vi "LedRingSubVI.vi"(8 "error in (no error)":errorcluster, 9 "Enum":enum16{"Idle", "Off", "Block", "Access"}(ring), 10 "VISA resource name in":refnum<visa-resource-name>, 11 "Boolean in":refnum<vi>) -> (0 "error out":errorcluster, 3 "VISA Refnum out":refnum<visa-resource-name>)   [LabVIEW 2024]
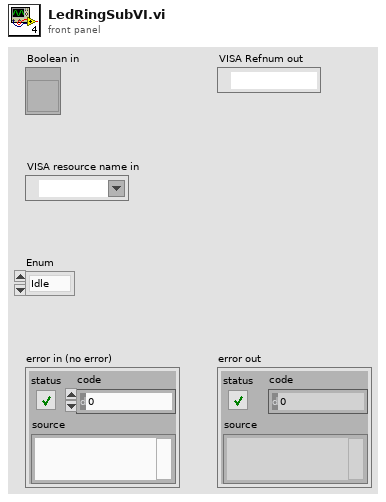
[diagram p1: front panel]
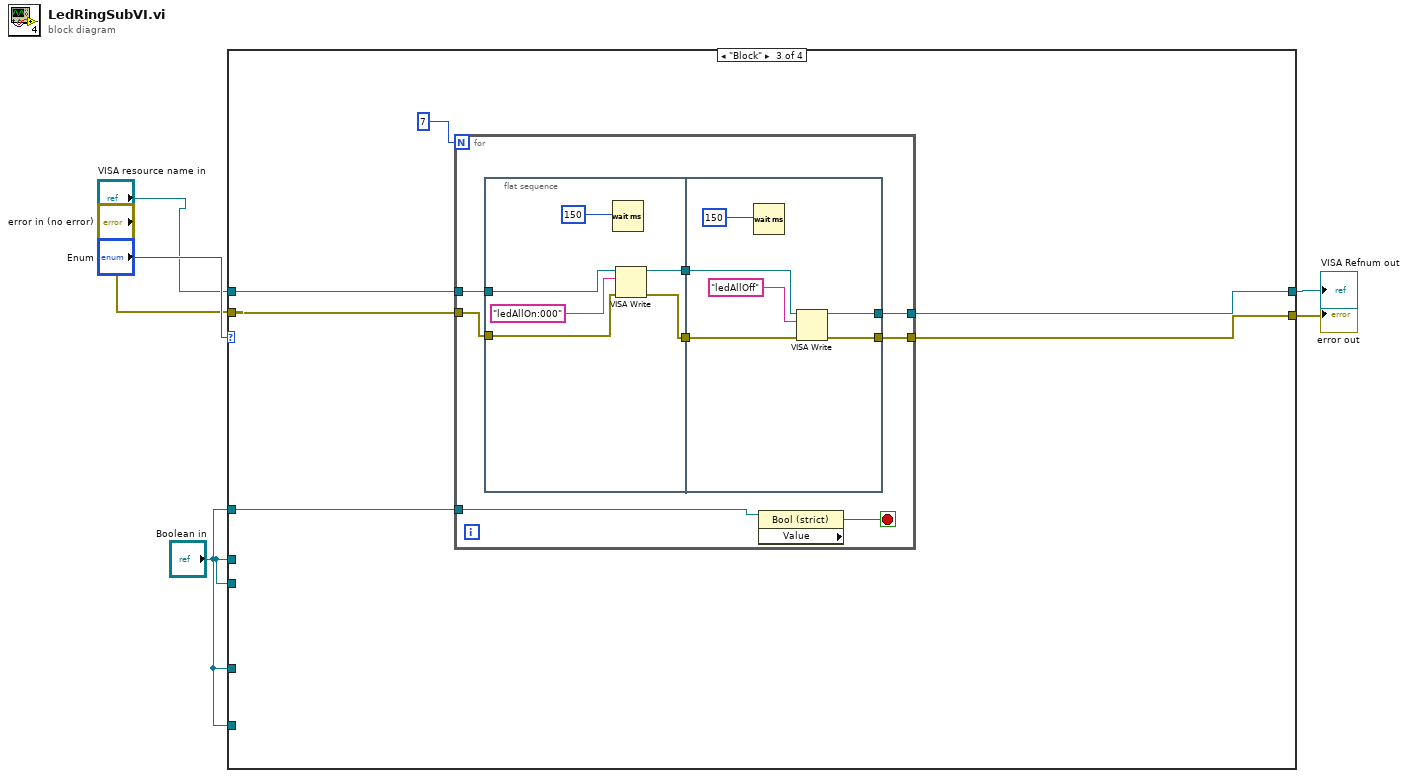
[diagram p0: block diagram]
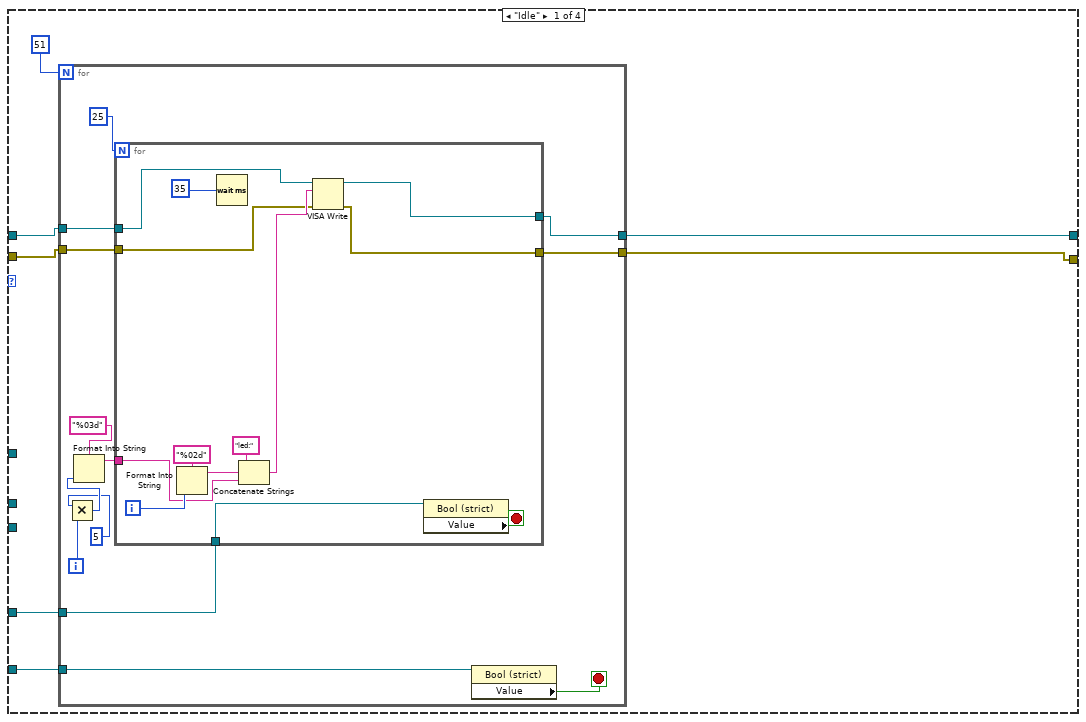
[diagram p2: hidden frame]
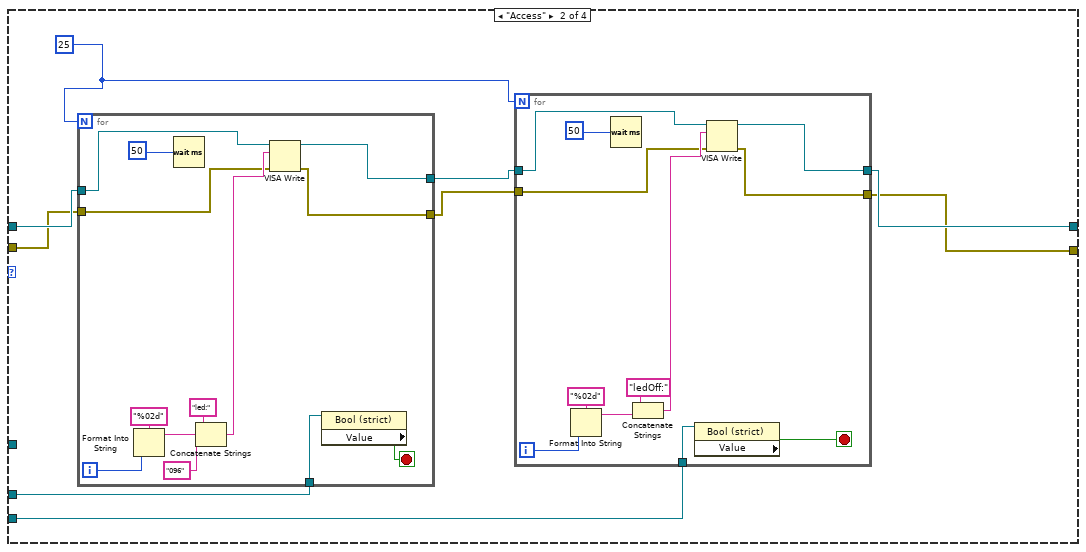
[diagram p3: hidden frame]
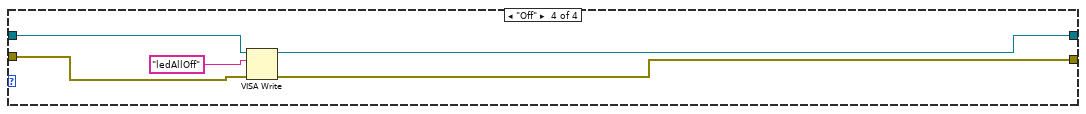
[diagram p4: hidden frame]
diagram:
  n1 = case shown="\"Access\"" "Enum" {
    tunnel: "VISA resource name in" -> [w12 w45 w78 w103]
    tunnel: "error in (no error)" -> [w13 w44 w77 w102]
    tunnel: [w10 w43 w76 w101] -> w5
    tunnel: [w9 w42 w75 w100] -> w4
    tunnel: "Boolean in" -> [w8 _ _ _]
    tunnel: "Boolean in" -> [w7 _ _ _]
    tunnel: "Boolean in" -> [_ w41 _ _]
    tunnel: "Boolean in" -> [_ w40 _ _]
    tunnel: "Boolean in" -> [_ _ w74 _]
    frame "Idle" {
      n2 = for {
        N: 51 -> [_]
        tunnel: w13 -> [w26]
        tunnel: w12 -> [w25]
        tunnel: [w21] -> w10
        tunnel: [w20] -> w9
        tunnel: w8 -> [w15]
        tunnel: w7 -> [w14]
        i -> [w19]
        stop <- w16 stop-if-true
        n3 = Multiply(x=5, y=w19) -> (x*y=w18:i32)
        n4 = Format Into String(format string="%03d", w18) -> (resulting string=w22:string)  [unwired: 2 in, 1 out]
        n5 = for {
          N: 25 -> [_]
          tunnel: w26 -> [w32]
          tunnel: w25 -> [w33]
          tunnel: [w34] -> w20
          tunnel: [w35] -> w21
          tunnel: w22 -> [w29]
          tunnel: w15 -> [w27]
          i -> [w38]
          stop <- w28 stop-if-true
          n6 = Format Into String(format string="%02d", w38) -> (resulting string=w30:string)  [unwired: 2 in, 1 out]
          n7 = Wait (ms)(milliseconds to wait=u32 35 ("millisecond multiple")) -> ()  [unwired: 1 out]
          n8 = Concatenate Strings("led:", w30, w29) -> (w36:string)
          n9 = VISA Write(VISA resource name=w33, write buffer=w36, error in (no error)=w32) -> (VISA resource name out=w35:refnum<visa-resource-name>, error out=w34:errorcluster)  [unwired: 1 out]
          n10 = property class="Bool (strict)"(reference=w27) -> ("Value"=w28:bool)  [unwired: 1 in, 2 out]
        }
        n11 = property class="Bool (strict)"(reference=w14) -> ("Value"=w16:bool)  [unwired: 1 in, 2 out]
      }
    }
    frame "Access" {
      w46 = 25
      n12 = for {
        N: w46 -> [_]
        tunnel: w44 -> [w65]
        tunnel: w45 -> [w66]
        tunnel: [w67] -> w47
        tunnel: [w68] -> w48
        tunnel: w41 -> [w61]
        i -> [w72]
        stop <- w62 stop-if-true
        n13 = Format Into String(format string="%02d", w72) -> (resulting string=w63:string)  [unwired: 2 in, 1 out]
        n14 = Wait (ms)(milliseconds to wait=u32 50 ("millisecond multiple")) -> ()  [unwired: 1 out]
        n15 = Concatenate Strings("led:", w63, "096") -> (w69:string)
        n16 = VISA Write(VISA resource name=w66, write buffer=w69, error in (no error)=w65) -> (VISA resource name out=w68:refnum<visa-resource-name>, error out=w67:errorcluster)  [unwired: 1 out]
        n17 = property class="Bool (strict)"(reference=w61) -> ("Value"=w62:bool)  [unwired: 1 in, 2 out]
      }
      n18 = for {
        N: w46 -> [_]
        tunnel: w47 -> [w53]
        tunnel: w48 -> [w54]
        tunnel: [w55] -> w42
        tunnel: [w56] -> w43
        tunnel: w40 -> [w49]
        i -> [w59]
        stop <- w50 stop-if-true
        n19 = Format Into String(format string="%02d", w59) -> (resulting string=w51:string)  [unwired: 2 in, 1 out]
        n20 = Wait (ms)(milliseconds to wait=u32 50 ("millisecond multiple")) -> ()  [unwired: 1 out]
        n21 = Concatenate Strings("ledOff:", w51) -> (w57:string)
        n22 = property class="Bool (strict)"(reference=w49) -> ("Value"=w50:bool)  [unwired: 1 in, 2 out]
        n23 = VISA Write(VISA resource name=w54, write buffer=w57, error in (no error)=w53) -> (VISA resource name out=w56:refnum<visa-resource-name>, error out=w55:errorcluster)  [unwired: 1 out]
      }
    }
    frame "Block" {
      n24 = for {
        N: 7 -> [_]
        tunnel: w78 -> [w85]
        tunnel: w77 -> [w84]
        tunnel: [w83] -> w76
        tunnel: [w82] -> w75
        tunnel: w74 -> [w80]
        stop <- w81 stop-if-true
        n25 = flat-sequence {
          tunnel: [w91] -> w87
          tunnel: [w90] -> w86
          tunnel: w85 -> [w89]
          tunnel: w84 -> [w88]
          tunnel: w87 -> [w98]
          tunnel: w86 -> [w97]
          tunnel: [w96] -> w83
          tunnel: [w95] -> w82
          frame #0 {
            n26 = Wait (ms)(milliseconds to wait=u32 150 ("millisecond multiple")) -> ()  [unwired: 1 out]
            n27 = VISA Write(VISA resource name=w89, write buffer="ledAllOn:000", error in (no error)=w88) -> (VISA resource name out=w91:refnum<visa-resource-name>, error out=w90:errorcluster)  [unwired: 1 out]
          }
          frame #1 {
            n28 = Wait (ms)(milliseconds to wait=u32 150 ("millisecond multiple")) -> ()  [unwired: 1 out]
            n29 = VISA Write(VISA resource name=w98, write buffer="ledAllOff", error in (no error)=w97) -> (VISA resource name out=w96:refnum<visa-resource-name>, error out=w95:errorcluster)  [unwired: 1 out]
          }
        }
        n30 = property class="Bool (strict)"(reference=w80) -> ("Value"=w81:bool)  [unwired: 1 in, 2 out]
      }
    }
    frame "Off" {
      n31 = VISA Write(VISA resource name=w103, write buffer="ledAllOff", error in (no error)=w102) -> (VISA resource name out=w101:refnum<visa-resource-name>, error out=w100:errorcluster)  [unwired: 1 out]
    }
  }
  "VISA Refnum out" <- w5
  "error out" <- w4
